vi "RSZVB Set Type Of Port Transfer Model.vi"(7 "Model Type (Linear Approximation)":i32(ring)=1 items=["Data Set", "Linear Approximation", "Electronic Attenuator Only", "None or Mechanical Attenuator"], 8 "error in (no error)":errorcluster {"code" format="%.0x"}, 9 "Port (1)":i32=1, 10 "Channel (1)":i32=1, 11 "VISA session":refnum<visa-resource-name>) -> (0 "error out":errorcluster {"code" format="%.0x"}, 3 "dup VISA session":refnum<visa-resource-name>)   [LabVIEW 2011]
doc: "This VI selects the type of advanced power transfer model for the converter port <Pt>.\n\nNote(s):This VI overwrites by the general power transfer model settings; see [SENSe<Ch>:]CONVerter:DESCription.\n\nRemote-control command(s):\nSOURce<Ch>:POWer<Pt>:CONVerter:TRANsfer:DESCription DSET | LAPProx"
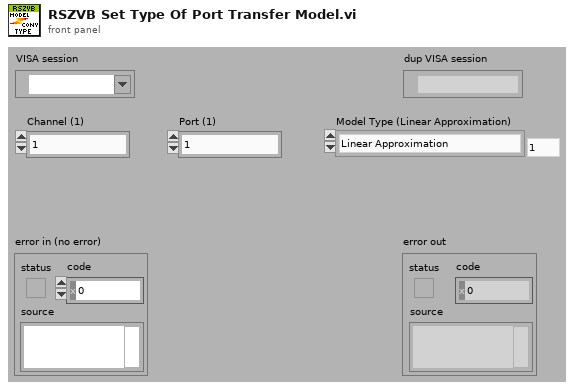
[diagram p1: front panel]
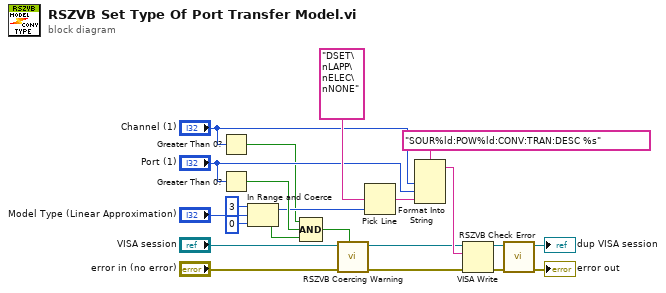
[diagram p0: block diagram]
diagram:
  n1 = Greater Than 0?(x="Channel (1)") -> (x > 0?=w3:bool)
  n2 = Greater Than 0?(x="Port (1)") -> (x > 0?=w18:bool)
  n3 = In Range and Coerce(upper limit=3, x="Model Type (Linear Approximation)", lower limit=0) -> (coerced(x)=w12:i32, In Range?=w17:bool)
  n4 = Compound Arithmetic op=AND(w3, w18, w17) -> (w19:bool)
  n5 = call "RSZVB Coercing Warning.vi"("In Range?"=w19, "error in (no error)"="error in (no error)", "VISA session"="VISA session") -> ("error out"=w14:errorcluster, "dup VISA session"=w13:refnum<visa-resource-name>)  [unwired: 7 in]
  n6 = Pick Line(multi-line string="DSET\nLAPP\nELEC\nNONE", line index=w12) -> (output string=w7:string)  [unwired: 1 in]
  n7 = Format Into String(format string="SOUR%ld:POW%ld:CONV:TRAN:DESC %s", "Channel (1)", "Port (1)", w7) -> (resulting string=w20:string)  [unwired: 2 in, 1 out]
  n8 = VISA Write(VISA resource name=w13, write buffer=w20, error in (no error)=w14) -> (VISA resource name out=w16:refnum<visa-resource-name>, error out=w15:errorcluster)  [unwired: 1 out]
  n9 = call "RSZVB Check Error.vi"("error in (no error)"=w15, "VISA session"=w16) -> ("error out"=→"error out":errorcluster, "dup VISA session"=→"dup VISA session":refnum<visa-resource-name>)  [unwired: 8 in]
